vi "Auto_Routine_LeaveRobotStartingZone.vi"(8 "error in (no error)":errorcluster) -> (0 "error out":errorcluster)   [LabVIEW 2023]
doc: "Leaves the community\n\ninput:\n--ErrorIn--\n\noutput:\n--ErrorOut--"
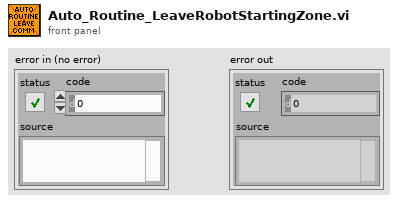
[diagram p1: front panel]
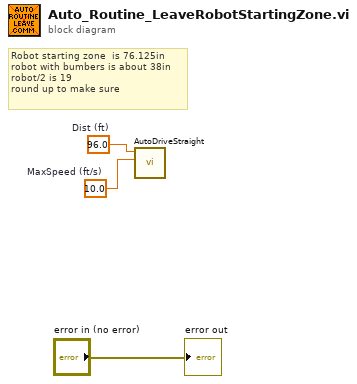
[diagram p0: block diagram]
diagram:
  w1 = 96.0  # Dist (ft)
  w2 = 10.0  # MaxSpeed (ft/s)
  # "Robot starting zone  is 76.125in \nrobot with bumbers is about 38in\nrobot/2 is 19\nround up to make sure"
  n1 = call "AutoDriveStraight.vi"("MaxSpeed (ft/s)"=w2, "Dist (ft)"=w1) -> ()  [unwired: 9 in, 1 out]
  "error out" <- "error in (no error)"
